vi "testComPort.vi"() -> ()   [LabVIEW 2016]
uses:
  ComPortActionTypeDef.ctl
panel:
  out "error out":errorcluster
  out "read buffer":string
  in  "VISA resource name":refnum<visa-resource-name>
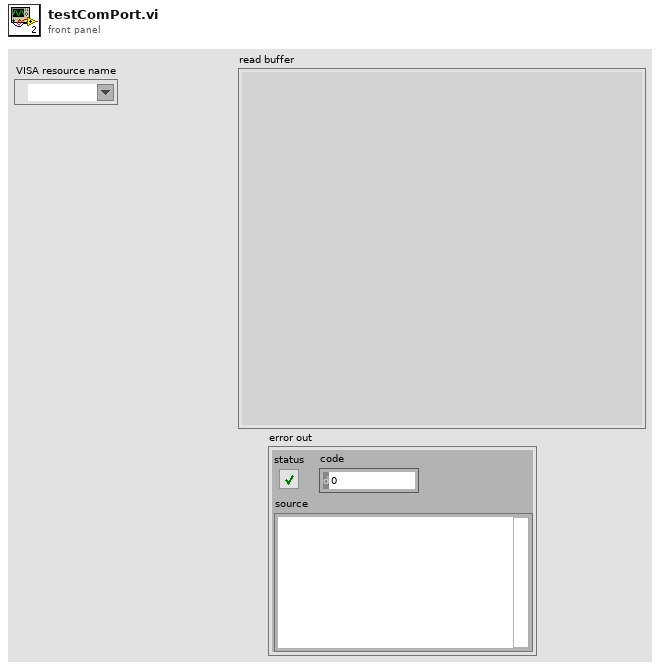
[diagram p1: front panel]
types:
  T1 = typedef "ComPortActionTypeDef.ctl" = enum16{"InitComPort", "ReadComPort", "WriteComePort", "CloseComPort"}
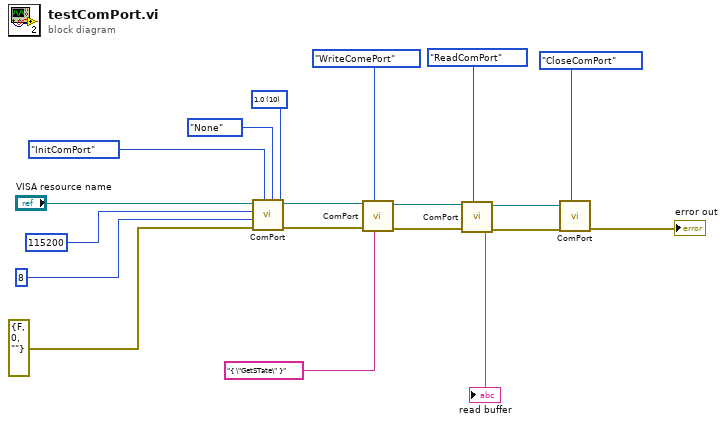
[diagram p0: block diagram]
diagram:
  w14 = u16 10 items=["1.0"=10, "1.5"=15, "2.0"=20] ("stop bits (10: 1 bit)")
  n1 = call "ComPort.vi"("stop bits (10: 1 bit)"=w14, "parity (0:none)"=enum16{"None", "Odd", "Even", "Mark", "Space"}."None", "ComAction"=ComPortActionTypeDef."InitComPort", "error in (no error)"=errorcluster {"status"=FALSE, "code"=0, "source"=""}, "data bits (8)"=u16 8, "baud rate (9600)"=u32 115200, "VISA resource name"="VISA resource name") -> ("error out"=w10:errorcluster, "VISA resource name out"=w13:refnum<visa-resource-name>)  [unwired: 2 in, 1 out]
  n2 = call "ComPort.vi"("write buffer"="{ \"GetSTate\" }", "ComAction"=ComPortActionTypeDef."WriteComePort", "error in (no error)"=w10, "VISA resource name"=w13) -> ("error out"=w9:errorcluster, "VISA resource name out"=w12:refnum<visa-resource-name>)  [unwired: 5 in, 1 out]
  n3 = call "ComPort.vi"("ComAction"=ComPortActionTypeDef."ReadComPort", "error in (no error)"=w9, "VISA resource name"=w12) -> ("error out"=w8:errorcluster, "VISA resource name out"=w11:refnum<visa-resource-name>, "read buffer"=→"read buffer":string)  [unwired: 6 in]
  n4 = call "ComPort.vi"("ComAction"=ComPortActionTypeDef."CloseComPort", "error in (no error)"=w8, "VISA resource name"=w11) -> ("error out"=→"error out":errorcluster)  [unwired: 6 in, 2 out]
